vi "Prototype.vi"() -> ()   [LabVIEW 2019]
uses:
  <vilib>/MagicBox/Device/Arduino/Arduino.lvclass
  <vilib>/MagicBox/Peripherals/POX/POX.lvclass
  <vilib>/MagicBox/Peripherals/POX/Read/Read Analog 1Smp 1Chl (Static, POX).vi
panel:
  out "error out":errorcluster
  out "POX Sample":string
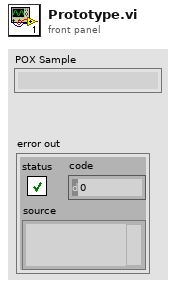
[diagram p1: front panel]
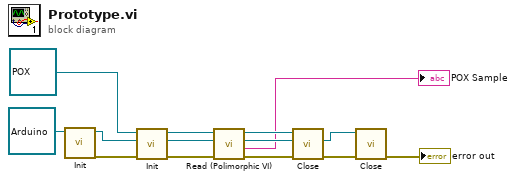
[diagram p0: block diagram]
diagram:
  n1 = call-dynamic "Init.vi"("Arduino in"=refnum<class "Arduino.lvclass"> refnum) -> ("error out"=w14:errorcluster, "Arduino out"=w9:refnum<class "Arduino.lvclass">)  [unwired: 9 in]
  n2 = call-dynamic "Init.vi"("error in (no error)"=w14, "Arduino in"=w9, "POX in"=refnum<class "POX.lvclass"> refnum) -> ("error out"=w13:errorcluster, "Arduino out"=w7:refnum<class "Arduino.lvclass">, "POX out"=w6:refnum<class "POX.lvclass">)  [unwired: 6 in]
  n3 = call-poly <vilib>:"Read (Polimorphic VI).vi"("error in (no error)"=w13, "Arduino in"=w7, "POX in"=w6) -> ("error out"=w12:errorcluster, "Read"=→"POX Sample":string, "Arduino out"=w5:refnum<class "Arduino.lvclass">, "POX out"=w4:refnum<class "POX.lvclass">)  [unwired: 5 in]
  n4 = call-dynamic "Close.vi"("error in (no error)"=w12, "Arduino in"=w5, "POX in"=w4) -> ("error out"=w11:errorcluster, "Arduino out"=w3:refnum<class "Arduino.lvclass">)  [unwired: 6 in, 1 out]
  n5 = call-dynamic "Close.vi"("error in (no error)"=w11, "Arduino in"=w3) -> ("error out"=→"error out":errorcluster)  [unwired: 8 in, 1 out]
